vi "Test data.vi"() -> ()   [LabVIEW 2013]
uses:
  Test Compiliation/Test Sector Cluster.ctl
panel:
  in  "Pixel Sectors":T1[](array[typedef])=array[48346 elements]
  out "Left Sector":u8
  out "Right Sector":u8
  in  "Sector Edges":u8[][](array[numeric])=[[26, 13], [26, 13], [26, 13], [26, 13], [26, 13], [27, 13], [27, 13], [27, 13], [27, 13], [27, 13], [27, 13], [27, 13], [27, 14], [27, 14], [27, 13], [26, 13], [26, 13], [26, 13], [26, 13], [26, 13], [26, 13], [26, 13], [26, 13], [26, 13], [26, 13], [26, 13], [26, 13], [26, 14], [26, 12], [26, 13], [26, 13], [26, 13], [26, 13], [26, 13], [26, 13], [26, 12], [26, 13], [26, 13], [26, 12], [26, 13], [26, 14], [26, 13], [26, 12], [26, 14], [26, 12], [26, 14], [26, 13], [26, 14], [26, 12], [26, 12], [26, 13], [26, 13], [26, 13], [26, 14], [26, 13], [26, 14], [26, 13], [26, 13], [26, 14], [26, 14], [26, 14], [26, 13], [26, 13], [26, 13], [26, 13], [26, 14], [26, 13], [26, 14], [26, 14], [26, 13], [26, 14], [26, 12], [26, 14], [26, 14], [26, 13], [26, 14], [26, 13], [26, 13], [26, 13], [26, 14], [26, 13], [26, 14], [26, 13], [26, 12], [26, 12], [26, 12], [26, 14], [26, 14], [26, 14], [26, 14], [26, 14], [26, 14], [26, 13], [26, 14], [26, 14], [26, 13], [26, 14], [26, 14], [26, 13], [26, 14], [26, 13], [26, 13], [26, 13], [26, 13], [26, 13], [26, 13], [26, 14], [26, 13], [26, 13], [26, 13], [26, 14], [26, 14], [26, 13], [26, 13], [26, 14], [26, 13], [27, 13], [27, 14], [27, 14], [27, 13], [27, 14], [27, 14], [27, 14], [27, 14], [26, 13], [26, 13], [27, 14], [27, 14], [27, 14], [27, 14], [27, 14], [26, 13], [26, 14], [26, 14], [26, 14], [26, 14], [26, 13], [26, 14], [26, 14], [26, 12], [26, 14], [26, 13], [26, 14], [26, 13], [26, 14], [27, 14], [26, 13], [26, 13], [26, 14], [26, 14], [26, 14], [26, 14], [26, 12], [26, 14], [26, 14], [27, 14], [26, 14], [27, 14], [26, 13], [26, 14], [26, 14], [26, 14], [26, 14], [27, 13], [26, 14], [27, 13], [26, 14], [26, 13], [26, 14], [26, 14], [26, 14], [26, 13], [26, 13], [26, 14], [26, 14], [26, 13], [26, 13], [26, 13], [26, 14], [26, 12], [27, 14], [26, 14], [26, 14], [26, 14], [26, 13], [26, 13], [26, 14], [26, 13], [26, 14], [26, 14], [26, 14], [26, 14], [26, 14], [27, 14], [26, 14], [26, 14], [26, 13], [27, 14], [26, 14], [26, 14], [26, 13], [27, 14], [26, 14], [26, 14], [26, 14], [26, 14], [26, 13], [26, 14], [27, 14], [27, 14], [26, 14], [26, 13], [26, 14], [26, 14], [27, 14], [27, 14], [26, 13], [26, 14], [26, 13], [26, 14], [26, 13], [27, 13], [26, 13], [27, 14], [27, 14], [27, 14], [27, 14], [26, 13], [26, 13], [27, 13], [26, 14], [26, 13], [26, 13], [26, 13], [27, 14], [26, 13], [27, 14], [26, 14], [27, 13], [27, 14], [27, 14], [27, 14], [26, 14], [26, 13], [27, 14], [26, 13], [27, 13], [27, 14], [27, 13], [27, 13], [27, 14], [26, 13], [27, 14], [26, 13], [27, 14], [26, 14], [27, 13], [27, 14], [27, 14], [27, 14], [27, 14], [26, 13], [27, 14], [27, 13], [27, 13], [27, 14], [27, 13], [26, 13], [27, 13], [27, 13], [27, 14], [27, 13], [27, 13], [27, 13], [27, 14], [27, 13], [27, 14], [27, 14], [27, 13], [27, 13], [27, 13], [27, 13], [27, 14], [27, 13], [27, 13], [27, 13], [27, 13], [27, 13], [27, 13], [27, 13], [27, 13], [27, 14], [27, 13], [27, 13], [27, 13], [27, 14], [27, 14], [27, 13], [27, 13], [27, 13], [27, 13], [27, 13], [27, 13], [27, 13], [27, 13], [27, 13], [27, 13], [27, 13], [27, 13], [27, 13], [27, 13], [27, 13], [27, 13], [27, 13], [27, 13], [27, 13], [27, 13], [26, 13], [27, 13], [26, 13], [27, 13], [26, 13], [26, 13], [26, 13], [27, 13], [26, 13], [26, 14], [26, 14], [26, 13], [27, 13], [27, 13], [27, 13], [26, 13], [27, 13], [26, 13], [27, 13], [27, 13], [27, 13], [27, 13], [26, 13], [27, 13], [27, 13], [27, 13], [27, 14], [26, 13], [27, 13], [27, 13], [27, 13], [27, 13], [27, 13], [27, 13], [27, 13], [26, 13], [27, 13], [26, 13], [26, 13], [26, 13], [26, 13], [26, 13], [26, 13], [26, 13], [27, 12], [27, 13], [27, 13], [27, 13], [27, 13], [26, 12], [27, 13], [26, 13], [27, 13], [27, 13], [27, 13], [27, 13], [27, 13], [27, 13], [27, 13], [27, 13], [27, 13], [28, 13], [27, 12], [27, 13], [27, 13], [28, 13], [27, 14], [27, 13], [27, 13], [27, 13], [27, 13], [27, 13], [27, 13], [27, 13], [27, 13], [27, 13], [27, 13], [27, 13], [27, 13], [27, 13], [27, 13], [26, 13], [27, 13], [27, 13], [27, 13], [27, 13], [27, 13], [27, 13], [26, 13], [27, 13], [27, 13], [27, 13], [26, 13], [27, 13], [27, 13], [27, 13], [26, 13], [27, 13], [26, 13], [27, 13], [27, 13], [27, 13], [27, 13], [27, 13], [27, 13], [27, 13], [27, 13], [27, 13], [27, 13], [27, 13], [27, 13], [27, 13], [27, 13], [26, 12], [27, 13], [27, 13], [26, 13], [27, 13], [26, 13], [27, 13], [27, 14], [27, 14], [26, 13], [27, 13], [27, 13], [27, 13], [27, 13], [27, 13], [27, 13], [27, 13], [27, 13], [27, 13], [27, 13], [27, 13], [27, 13], [27, 13], [27, 13], [27, 13], [27, 13], [27, 13], [27, 13], [27, 13], [27, 13], [27, 13], [27, 13], [27, 13], [27, 13], [27, 13], [27, 13], [27, 13], [27, 13], [27, 13], [27, 13], [27, 13], [27, 13], [27, 13], [27, 13], [27, 13], [27, 13], [27, 13], [27, 13], [27, 13], [27, 13], [27, 13], [27, 13], [27, 13], [28, 14], [28, 14], [28, 13], [27, 13], [27, 13], [27, 13], [27, 13], [27, 13], [27, 13], [27, 13], [27, 13], [27, 13], [27, 13], [27, 13], [27, 13], [27, 13], [27, 13]]
  in  "Right ROI":T2={"Global Rectangle"=[652, 103, 1033, 747], "Contours"=[{"ID"=enum."External", "Type"=7, "Coordinates"=[653, 483, 320, 379, 316305, 90000]}]} {"Contours"."Type" items=["No Selection", "Point", "Line", "Rectangle", "Oval", "Polygon", "Freehand Region", "Annulus", "Unused2", "Unused3", "Broken Line", "Freehand Line", "Rotated Rectangle"]}
  in  "Left ROI":T2={"Global Rectangle"=[158, 97, 539, 747], "Contours"=[{"ID"=enum."External", "Type"=7, "Coordinates"=[537, 477, 320, 379, 90000, 225000]}]} {"Contours"."Type" items=["No Selection", "Point", "Line", "Rectangle", "Oval", "Polygon", "Freehand Region", "Annulus", "Unused2", "Unused3", "Broken Line", "Freehand Line", "Rotated Rectangle"]}
  out "error out":errorcluster
  out "Image":T3(plugin-control)
  out "Frame #":i32
  in  "Frame":i32(c297)
  in  "stop":bool
  in  "Path":path=path "C:/Users/achiu/Documents/Projects - Current/HHMI - WBA/Support Files/Video/500Frames.avi"
  out "Right Wingbeat Avg Graph":u8[](graph)
  out "Left Wingbeat Avg Graph":u8[](graph)
  in  "[Average Sector Data]":u8[][](array[numeric])=array500x32[16000 elements]
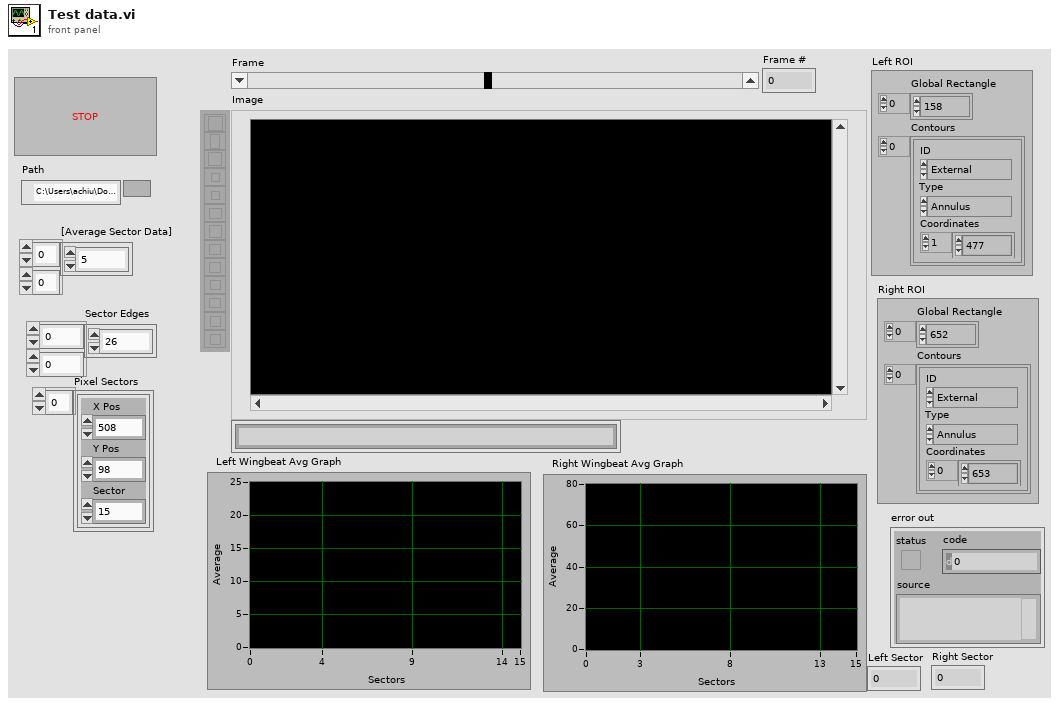
[diagram p1: front panel]
types:
  T1 = typedef "Test Sector Cluster.ctl" = cluster{"X Pos":u16, "Y Pos":u16, "Sector":u8}
  T2 = typedef "ROI Descriptor" = cluster{"Global Rectangle":i32[], "Contours":cluster{"ID":enum32{"External", "Internal"}, "Type":u32, "Coordinates":i32[]}[]}
  T3 = typedef "IMAQ Image.ctl" = refnum<image>
  T4 = typedef "Image Type" = u32
  T5 = typedef "IMAQ AVI2 Refnum.ctl" = refnum<k20>
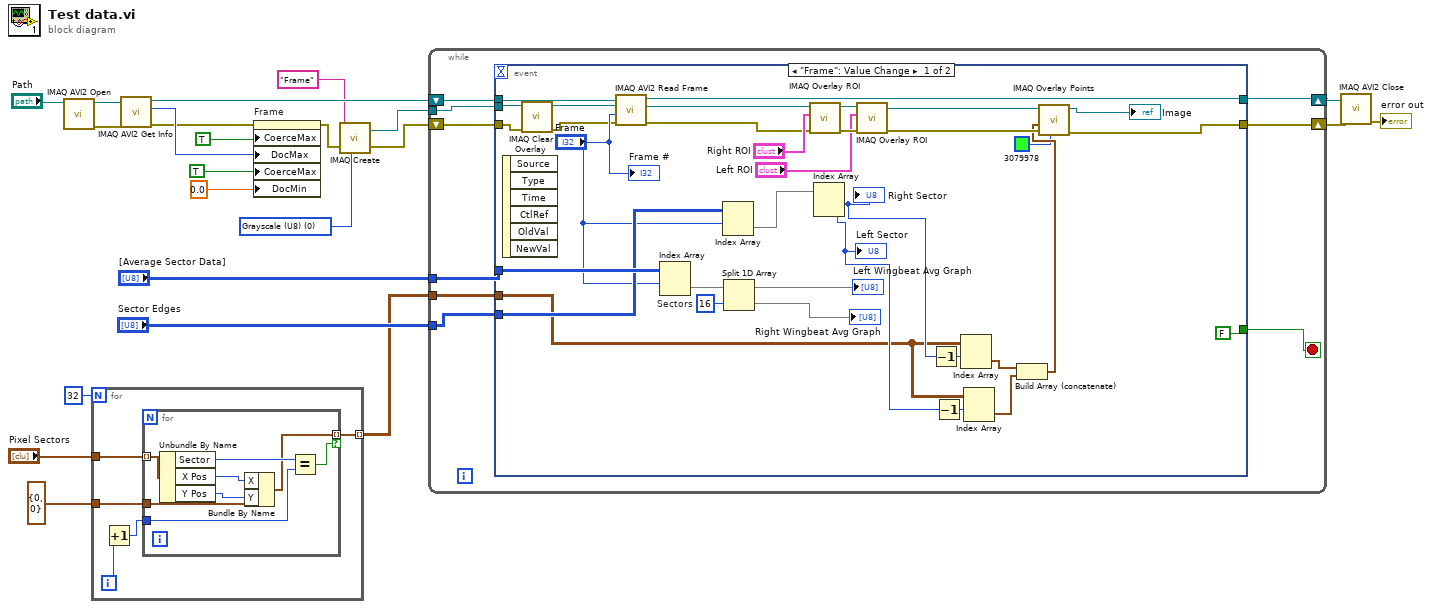
[diagram p0: block diagram]
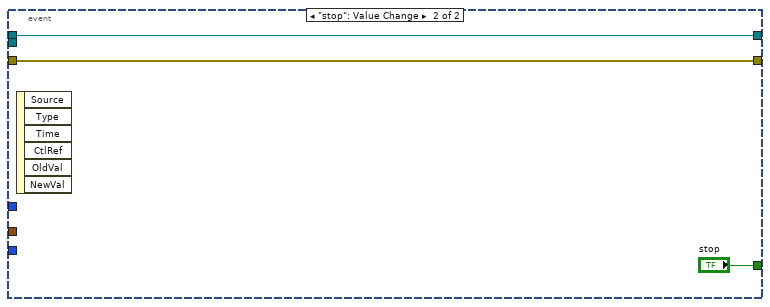
[diagram p2: hidden frame]
diagram:
  w10 = T4 0 items=["Grayscale (U8)", "Grayscale (I16)", "Grayscale (SGL)", "Complex (CSG)", "RGB (U32)", "HSL (U32)", "RGB (U64)", "Grayscale (U16)"] ("Image Type")
  n1 = call "IMAQ AVI2 Open"("AVI File Path"="Path") -> ("error out"=w22:errorcluster, "AVI Refnum"=w21:T5)  [unwired: 9 in]
  n2 = for {
    N: 32 -> [_]
    tunnel: "Pixel Sectors" -> [w28]
    tunnel: [w25] -> w1 mode=indexing
    tunnel: cluster{"X":i32, "Y":i32} {"X"=0, "Y"=0} ("Point Coordinates") -> [w24]
    i -> [w27]
    n3 = Increment(x=w27) -> (x+1=w26:i32)
    n4 = for {
      tunnel: w28 -> [w34] mode=indexing
      tunnel: w26 -> [w35]
      tunnel: [w29] -> w25 mode=indexing if=w33
      tunnel: w24 -> [w32]
      n5 = Unbundle By Name(w34) -> ("Sector"=w36:u8, "X Pos"=w31:u16, "Y Pos"=w30:u16)
      n6 = Bundle By Name(cluster=w32, "X"=w31, "Y"=w30) -> (w29:cluster{"X":i32, "Y":i32})
      n7 = Equal?(x=w36, y=w35) -> (x = y?=w33:bool)
    }
  }
  n8 = call "IMAQ AVI2 Get Info"("error in (no error)"=w22, "AVI Refnum"=w21) -> ("error out"=w18:errorcluster, "Number of Frames"=w19:u32, "AVI Refnum (duplicate)"=w17:T5)  [unwired: 5 in, 2 out]
  n9 = property on="Frame" class="Scroll (strict)"(error in=w18, "CoerceMax"=TRUE ("Coerce Maximum Value"), "DocMax"=w19, "CoerceMax"=TRUE ("Coerce Maximum Value"), "DocMin"=0.0 ("Doc Min")) -> (error out=w13:errorcluster)  [unwired: 1 in, 1 out]
  n10 = call "IMAQ Create"("Image Name"="Frame", "Image Type"=w10, "error in (no error)"=w13) -> ("New Image"=w9:T3, "error out"=w12:errorcluster)  [unwired: 2 in]
  n11 = while {
    shift-right: [w40] -> w8
    shift-left: w12 -> [w44]
    tunnel: "[Average Sector Data]" -> [w45]
    tunnel: w9 -> [w42]
    shift-right: [w41] -> w7
    shift-left: w17 -> [w43]
    tunnel: "Sector Edges" -> [w39]
    tunnel: w1 -> [w37]
    stop <- w38 stop-if-true
    n12 = event shown="[0] \"Frame\": Value Change" {
      selector: _ -> [_ _]
      dyn-events: _ -> [_ _]
      timeout: _ -> [_ _]
      tunnel: w45 -> [w79 _]
      tunnel: w44 -> [w49 w80]
      tunnel: w43 -> [w75 w81]
      tunnel: w42 -> [w50 _]
      tunnel: [w74 w81] -> w41
      tunnel: [w51 w80] -> w40
      tunnel: w39 -> [w67 _]
      tunnel: [FALSE ("stop") "stop"] -> w38
      tunnel: w37 -> [w58 _]
      event "Frame": Value Change {
        w65 = 16  # Sectors
        n13 = event-data() -> ()  [unwired: 1 in, 6 out]
        n14 = call "IMAQ Clear Overlay"("error in (no error)"=w49, "Image"=w50) -> ("error out"=w47:errorcluster, "Image Out"=w48:T3)  [unwired: 8 in]
        n15 = call "IMAQ AVI2 Read Frame"("error in (no error)"=w47, "Frame Number"="Frame", "Image"=w48, "AVI Refnum"=w75) -> ("error out"=w68:errorcluster, "Image Out"=w73:T3, "AVI Refnum (duplicate)"=w74:T5)  [unwired: 5 in]
        n16 = Index Array(array=w79, index (row)="Frame") -> (element=w78:u8[])  [unwired: 1 in]
        n17 = Index Array(array=w67, index (row)="Frame") -> (element=w63:u8[])  [unwired: 1 in]
        n18 = Split 1D Array(array=w78, index=w65) -> (first subarray=→"Left Wingbeat Avg Graph":u8[], second subarray=→"Right Wingbeat Avg Graph":u8[])
        n19 = call "IMAQ Overlay ROI"("error in (no error)"=w68, "ROI Descriptor"="Right ROI", "Image"=w73) -> ("error out"=w71:errorcluster, "Image Out"=w70:T3)  [unwired: 7 in]
        n20 = Index Array(array=w63) -> (element #1=w62:u8, element #2=w59:u8)  [unwired: 2 in]
        "Right Sector" <- w62
        "Left Sector" <- w59
        n21 = call "IMAQ Overlay ROI"("error in (no error)"=w71, "ROI Descriptor"="Left ROI", "Image"=w70) -> ("error out"=w57:errorcluster, "Image Out"=w56:T3)  [unwired: 7 in]
        n22 = Decrement(x=w62) -> (x-1=w61:u8)
        n23 = Decrement(x=w59) -> (x-1=w60:u8)
        n24 = Index Array(array=w58, index (row)=w61) -> (element=w55:cluster{"X":i32, "Y":i32}[])  [unwired: 1 in]
        n25 = Index Array(array=w58, index (row)=w60) -> (element=w54:cluster{"X":i32, "Y":i32}[])  [unwired: 1 in]
        n26 = Build Array (concatenate)(w55, w54) -> (w53:cluster{"X":i32, "Y":i32}[])
        n27 = call "IMAQ Overlay Points"("Color"=u32 3079978, "error in (no error)"=w57, "Array of Points"=w53, "Image"=w56) -> ("error out"=w51:errorcluster, "Image Out"=→"Image":T3)  [unwired: 6 in]
        "Frame #" <- "Frame"
      }
      event "stop": Value Change {
        n28 = event-data() -> ()  [unwired: 1 in, 6 out]
      }
    }
  }
  n29 = call "IMAQ AVI2 Close"("error in (no error)"=w8, "AVI Refnum"=w7) -> ("error out"=→"error out":errorcluster)  [unwired: 9 in]
